vi "EventBuilder.contents.vi"() -> ()   [LabVIEW 2014, in "EventBuilder.lvlib"]
doc: "loads all VIs into memory - required for building an application"
uses:
  EventBuilder.lvlib
panel:
  out "error out":errorcluster
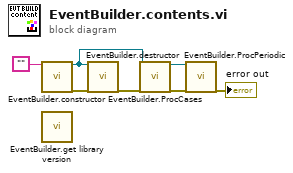
[diagram p0: block diagram]
diagram:
  n1 = call "EventBuilder.constructor.vi"("name"="") -> ("i ref out"=w5:refnum<vi>, "error out"=w4:errorcluster)  [unwired: 16 in, 1 out]
  n2 = call "EventBuilder.get library version.vi"() -> ()  [unwired: 1 in, 1 out]
  n3 = call "EventBuilder.destructor.vi"("i ref in"=w5, "error in (no error)"=w4) -> ("error out"=w3:errorcluster)  [unwired: 17 in]
  n4 = call "EventBuilder.ProcCases.vi"("i ref in"=w5, "error in (no error)"=w3) -> ("i ref out"=w6:refnum<vi>, "error out"=w2:errorcluster)  [unwired: 15 in, 1 out]
  n5 = call "EventBuilder.ProcPeriodic.vi"("i ref in"=w6, "error in (no error)"=w2) -> ("error out"=→"error out":errorcluster)  [unwired: 15 in, 2 out]
